vi "Init.vi"(3 "Container State":T3, 4 "Previous State":variant, 5 "Previous Version":T2) -> (2 "Current State":T1={"Pin Disabled?"=[enum."Enabled", enum."Enabled", enum."Enabled", enum."Enabled", enum."Enabled", enum."Enabled", enum."Enabled", enum."Enabled", enum."Enabled", enum."Enabled", enum."Enabled", enum."Enabled", enum."Enabled", enum."Enabled", enum."Enabled", enum."Enabled", enum."Enabled", enum."Enabled", enum."Enabled", enum."Enabled"], "Pin Name"=["", "", "", "", "", "", "", "", "", "", "", "", "", "", "", "", "", "", "", ""], "Pin ID"=["0", "1", "2", "3", "4", "5", "6", "7", "8", "9", "10", "11", "12", "13", "14", "15", "16", "17", "18", "19"], "Connector Name"="", "Row Name 1"="", "Row Name 2"=""})   [LabVIEW 2021, in "roboRIO 4 Bank.xctl"]
uses:
  <vilib>/myRIO/Common/Instrument Driver Framework/Utilities/xctls/roboRIO 4 Bank/roboRIO 4 Bank.xctl
  <vilib>/_xctls/Container State.ctl
  <vilib>/_xctls/Version.ctl
  <vilib>/myRIO/Common/Instrument Driver Framework/Utilities/xctls/roboRIO 4 Bank/State.ctl
  <vilib>/_xctls/XControlSupport.lvlib
panel:
  in  "Default Control State":T1={"Pin Disabled?"=[enum."Enabled", enum."Enabled", enum."Enabled", enum."Enabled", enum."Enabled", enum."Enabled", enum."Enabled", enum."Enabled", enum."Enabled", enum."Enabled", enum."Enabled", enum."Enabled", enum."Enabled", enum."Enabled", enum."Enabled", enum."Enabled", enum."Enabled", enum."Enabled", enum."Enabled", enum."Enabled"], "Pin Name"=["", "", "", "", "", "", "", "", "", "", "", "", "", "", "", "", "", "", "", ""], "Pin ID"=["0", "1", "2", "3", "4", "5", "6", "7", "8", "9", "10", "11", "12", "13", "14", "15", "16", "17", "18", "19"], "Connector Name"="", "Row Name 1"="", "Row Name 2"=""}
  in  "Default Indicator State":T1={"Pin Disabled?"=[enum."Enabled", enum."Enabled", enum."Enabled", enum."Enabled", enum."Enabled", enum."Enabled", enum."Enabled", enum."Enabled", enum."Enabled", enum."Enabled", enum."Enabled", enum."Enabled", enum."Enabled", enum."Enabled", enum."Enabled", enum."Enabled", enum."Enabled", enum."Enabled", enum."Enabled", enum."Enabled"], "Pin Name"=["", "", "", "", "", "", "", "", "", "", "", "", "", "", "", "", "", "", "", ""], "Pin ID"=["0", "1", "2", "3", "4", "5", "6", "7", "8", "9", "10", "11", "12", "13", "14", "15", "16", "17", "18", "19"], "Connector Name"="", "Row Name 1"="", "Row Name 2"=""}
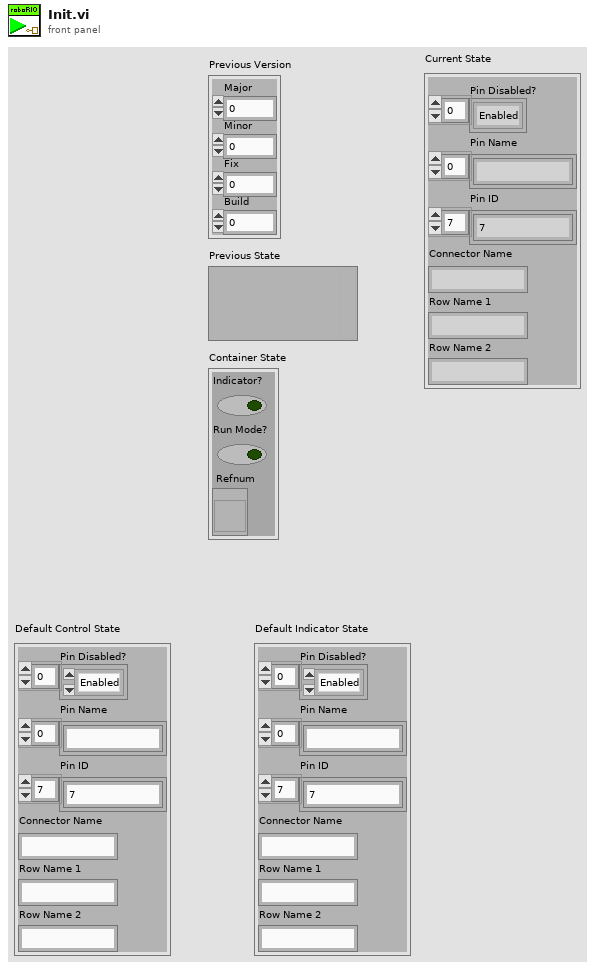
[diagram p1: front panel]
types:
  T1 = typedef "roboRIO 4 Bank.xctl/State.ctl" = cluster{"Pin Disabled?":enum8{"Enabled", "Disabled", "Disabled and Grayed Out"}[], "Pin Name":string[], "Pin ID":string[], "Connector Name":string, "Row Name 1":string, "Row Name 2":string}
  T2 = typedef "XControlSupport.lvlib/Version.ctl" = cluster{"Major":u16, "Minor":u16, "Fix":u16, "Build":u16}
  T3 = typedef "XControlSupport.lvlib/Container State.ctl" = cluster{"Indicator?":bool, "Run Mode?":bool, " Refnum":refnum<vi>}
  T4 = enum8{"Enabled", "Disabled", "Disabled and Grayed Out"}[]
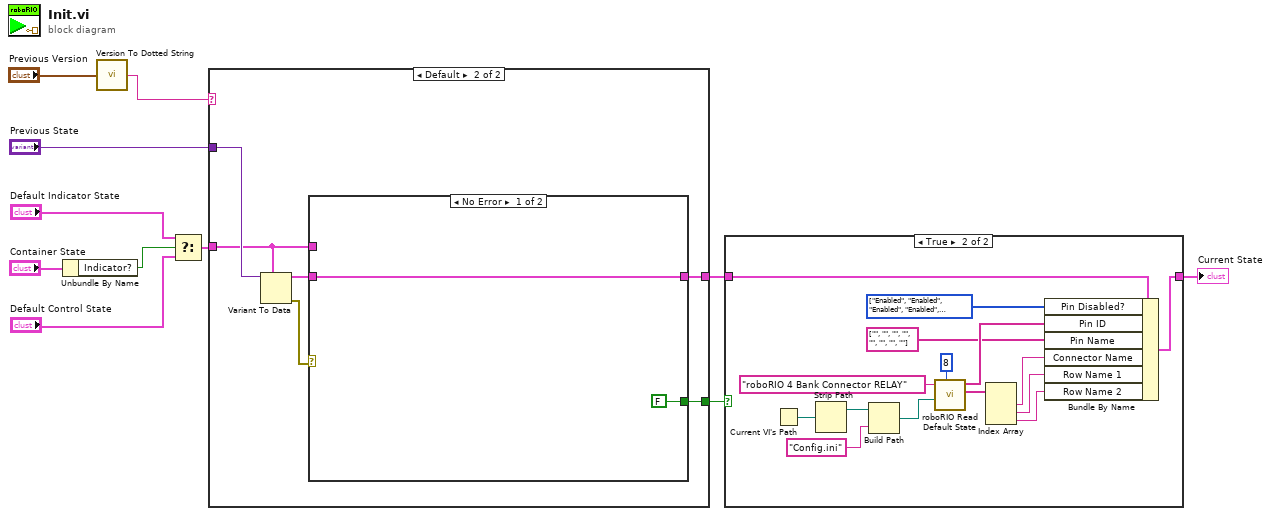
[diagram p0: block diagram]
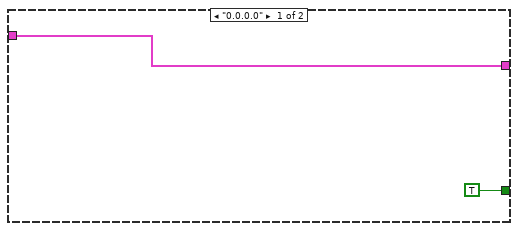
[diagram p3: hidden frame]
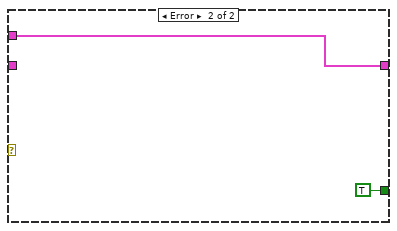
[diagram p4: hidden frame]
diagram:
  n1 = Unbundle By Name("Container State") -> ("Indicator?"=w9:bool)
  n2 = call <vilib>:"Version To Dotted String.vi"("Version"="Previous Version") -> ("String Version"=w6:string)
  n3 = Select(t="Default Indicator State", s=w9, f="Default Control State") -> (s? t:f=w8:T1)
  n4 = case shown="Default" w6 {
    tunnel: "Previous State" -> [_ w19]
    tunnel: [w13 w15] -> w4
    tunnel: w8 -> [w13 w16]
    tunnel: [TRUE w14] -> w5
    frame "0.0.0.0" {
    }
    frame Default {
      n5 = Variant To Data(type=w16, Variant=w19) -> (data=w17:T1, error out=w18:errorcluster)  [unwired: 1 in]
      n6 = case shown="No Error" w18 {
        tunnel: w17 -> [w21 _]
        tunnel: [w21 w22] -> w15
        tunnel: w16 -> [_ w22]
        tunnel: [FALSE TRUE] -> w14
        frame No Error {
        }
        frame Error {
        }
      }
    }
  }
  n7 = case shown="True" w5 {
    tunnel: [w24 w27] -> w3
    tunnel: w4 -> [w24 w28]
    frame False {
    }
    frame True {
      w26 = T4 [enum."Enabled", enum."Enabled", enum."Enabled", enum."Enabled", enum."Enabled", enum."Enabled", enum."Enabled", enum."Enabled"] items=["Enabled", "Disabled", "Disabled and Grayed Out"] ("subarray")
      n8 = Current VI's Path() -> (path=w37:path)
      n9 = Strip Path(path=w37) -> (stripped path=w38:path)  [unwired: 1 out]
      n10 = Build Path(base path=w38, name or relative path="Config.ini") -> (appended path=w34:path)
      n11 = call <vilib>:"roboRIO Read Default State.vi"("Size"=8, "Path"=w34, "Connector"="roboRIO 4 Bank Connector RELAY") -> ("Default Connector Info"=w32:string[], "Default Pins IDs"=w33:string[])  [unwired: 6 in, 1 out]
      n12 = Index Array(array=w32) -> (element #1=w31:string, element #2=w30:string, element #3=w29:string)  [unwired: 3 in]
      n13 = Bundle By Name(cluster=w28, "Pin Disabled?"=w26, "Pin ID"=w33, "Pin Name"=string[] ["", "", "", "", "", "", "", ""] ("Pin Alias"), "Connector Name"=w31, "Row Name 1"=w30, "Row Name 2"=w29) -> (w27:T1)
    }
  }
  "Current State" <- w3
